vi "Single Channel Temperature Log with Header.vi"() -> ()   [LabVIEW 2012]
doc: "This VI acquires temperature values every second. This VI also takes a running average of the last five temperature measurements and displays both the raw data and the running average in the strip chart. This VI also logs the raw data to a text file."
panel:
  in  "Stop Button":bool
  out "Temperature History":cluster{dbl, "Temperature Value":dbl}(graph)
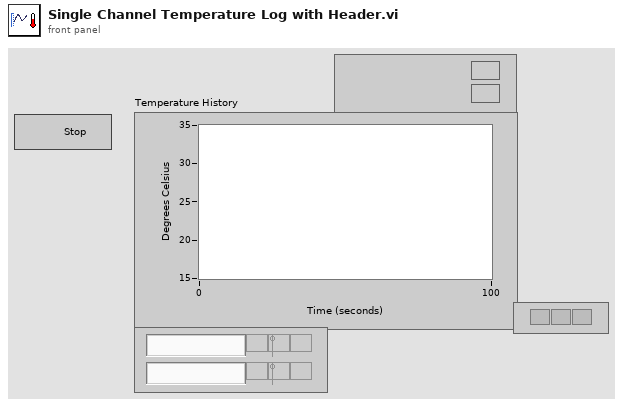
[diagram p1: front panel]
types:
  T1 = enum16{"open", "replace", "create", "open or create", "replace or create", "replace or create with confirmation"}
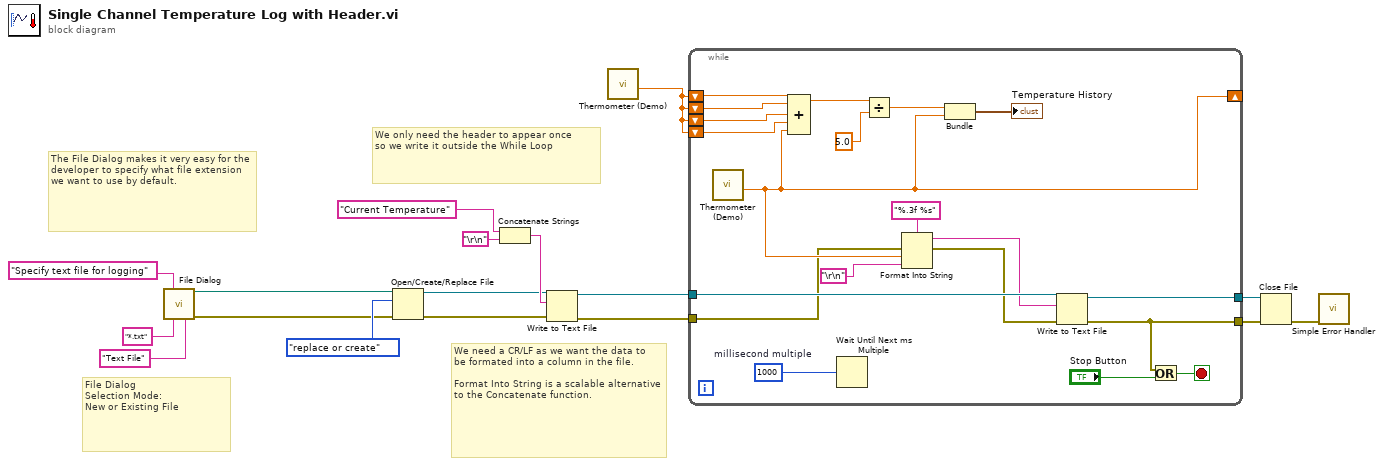
[diagram p0: block diagram]
diagram:
  # "File Dialog \nSelection Mode:\nNew or Existing File"
  # "We need a CR/LF as we want the data to\nbe formated into a column in the file.\n\nFormat Into String is a scalable alternative to the Concatenate function."
  # "We only need the header to appear once\nso we write it outside the While Loop"
  # "The File Dialog makes it very easy for the developer to specify what file extension we want to use by default."
  n1 = call "File Dialog"("prompt"="Specify text file for logging" ("pattern label"), "pattern (all files)"="*.txt", "pattern label"="Text File") -> ("selected path"=w7:path, "error out"=w1:errorcluster)  [unwired: 9 in, 2 out]
  n2 = Open/Create/Replace File(file path (use dialog)=w7, error in=w1, operation (0:open)=T1."replace or create") -> (refnum out=w10:refnum<file>, error out=w11:errorcluster)  [unwired: 4 out]
  n3 = Concatenate Strings("Current Temperature" ("string"), "\r\n" ("End of Line Constant")) -> (w12:string)
  n4 = Write to Text File(file (use dialog)=w10, text=w12, error in=w11) -> (refnum out=w4:refnum<file>, error out=w3:errorcluster)  [unwired: 2 out]
  n5 = call "Thermometer (Demo).vi"() -> ("Temperature Value"=w17:dbl)  [unwired: 11 in]
  n6 = while {
    shift-right: [w23] -> _
    shift-left: w17 -> [w36]
    shift-left: w17 -> [w35]
    shift-left: w17 -> [w32]
    shift-left: w17 -> [w31]
    tunnel: w3 -> [w21]
    tunnel: [w26] -> w15
    tunnel: w4 -> [w28]
    tunnel: [w27] -> w14
    stop <- w24 stop-if-true
    w37 = u32 1000  # millisecond multiple
    n7 = call "Thermometer (Demo).vi"() -> ("Temperature Value"=w23:dbl)  [unwired: 11 in]
    n8 = Compound Arithmetic op=ADD(w36, w35, w32, w31, w23) -> (w34:dbl)
    n9 = Wait Until Next ms Multiple(millisecond multiple=w37) -> ()  [unwired: 1 out]
    n10 = Divide(x=w34, y=5.0) -> (x/y=w30:dbl)
    n11 = Format Into String "Format Into String"(format string="%.3f %s", error in=w21, w23, "\r\n") -> (resulting string=w22:string, error out=w20:errorcluster)  [unwired: 1 in]
    n12 = Bundle(w30, "Temperature Value"=w23) -> (→"Temperature History":cluster{dbl, "Temperature Value":dbl})  [unwired: 1 in]
    n13 = Write to Text File(file (use dialog)=w28, text=w22, error in=w20) -> (refnum out=w27:refnum<file>, error out=w26:errorcluster)  [unwired: 2 out]
    n14 = Or(x=w26, y="Stop Button") -> (x .or. y?=w24:bool)
  }
  n15 = Close File(refnum=w14, error in=w15) -> (error out=w16:errorcluster)  [unwired: 1 out]
  n16 = call <vilib>:"Simple Error Handler.vi"("error in (no error)"=w16) -> ()  [unwired: 1 in, 8 out]
